vi "Joystick Get.vi"() -> (0 "Raw Joystick 2 Data":T2, 1 "Raw Joystick 1 Data":T2, 3 "Mapped Data":T3)   [LabVIEW 2013]
uses:
  Joystick Data.ctl
  <vilib>/Rock Robotics/WPI/Joystick/WPI_JoystickButtonState.ctl
  <vilib>/Rock Robotics/WPI/Joystick/WPI_JoystickGetSetRefNum.vi
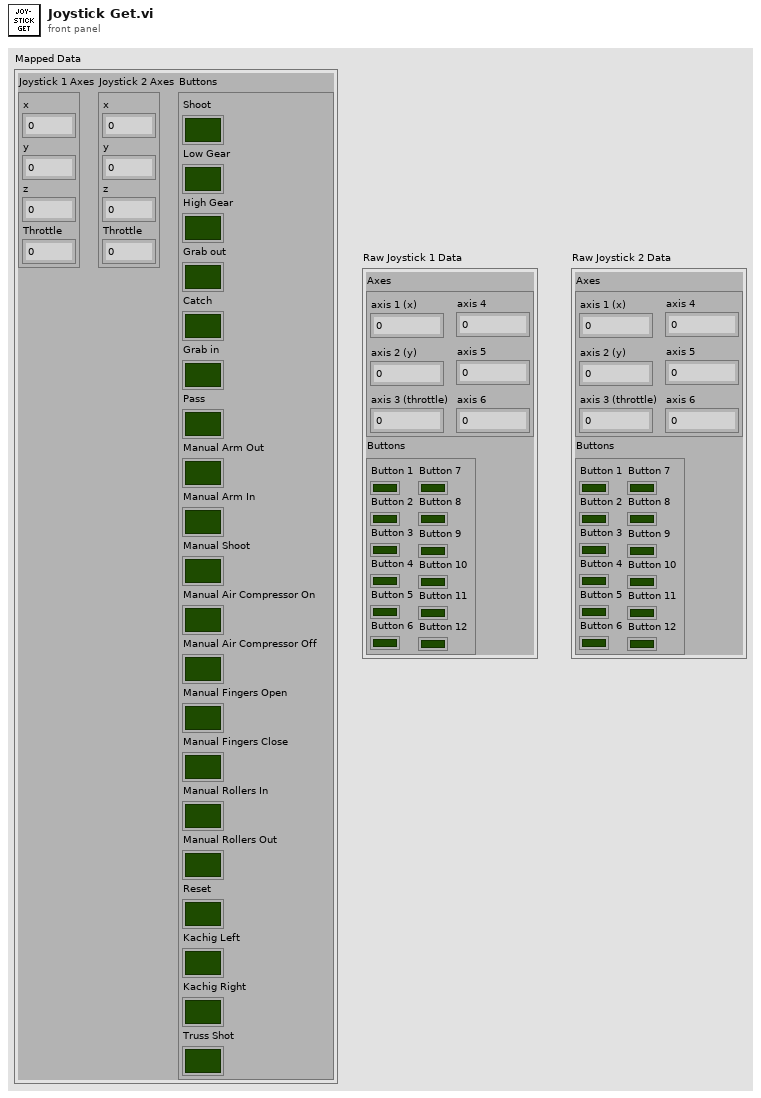
[diagram p1: front panel]
types:
  T1 = typedef "WPI_JoystickButtonState.ctl" = cluster{"Button 1":bool, "Button 2":bool, "Button 3":bool, "Button 4":bool, "Button 5":bool, "Button 6":bool, "Button 7":bool, "Button 8":bool, "Button 9":bool, "Button 10":bool, "Button 11":bool, "Button 12":bool}
  T2 = cluster{"Axes":cluster{"axis 1 (x)":dbl, "axis 2 (y)":dbl, "axis 3 (throttle)":dbl, "axis 4":dbl, "axis 5":dbl, "axis 6":dbl}, "Buttons":T1}
  T3 = typedef "Joystick Data.ctl" = cluster{"Joystick 1 Axes":cluster{"x":dbl, "y":dbl, "z":dbl, "Throttle":dbl}, "Joystick 2 Axes":cluster{"x":dbl, "y":dbl, "z":dbl, "Throttle":dbl}, "Buttons":cluster{"Shoot":bool, "Low Gear":bool, "High Gear":bool, "Grab out":bool, "Catch":bool, "Grab in":bool, "Pass":bool, "Manual Arm Out":bool, "Manual Arm In":bool, "Manual Shoot":bool, "Manual Air Compressor On":bool, "Manual Air Compressor Off":bool, "Manual Fingers Open":bool, "Manual Fingers Close":bool, "Manual Rollers In":bool, "Manual Rollers Out":bool, "Reset":bool, "Kachig Left":bool, "Kachig Right":bool, "Truss Shot":bool}}
  T4 = typedef "WPI_JoystickDevRef.ctl" = cluster{"Device":T5}
  T5 = typedef "WPI_JoystickDeviceEnum.ctl" = enum16{"USB 1", "USB 2", "USB 3", "USB 4", "Kinect 1", "Kinect 2"}
  T6 = cluster{"axis 1 (x)":dbl, "axis 2 (y)":dbl, "axis 3 (throttle)":dbl, "axis 4":dbl, "axis 5":dbl, "axis 6":dbl}
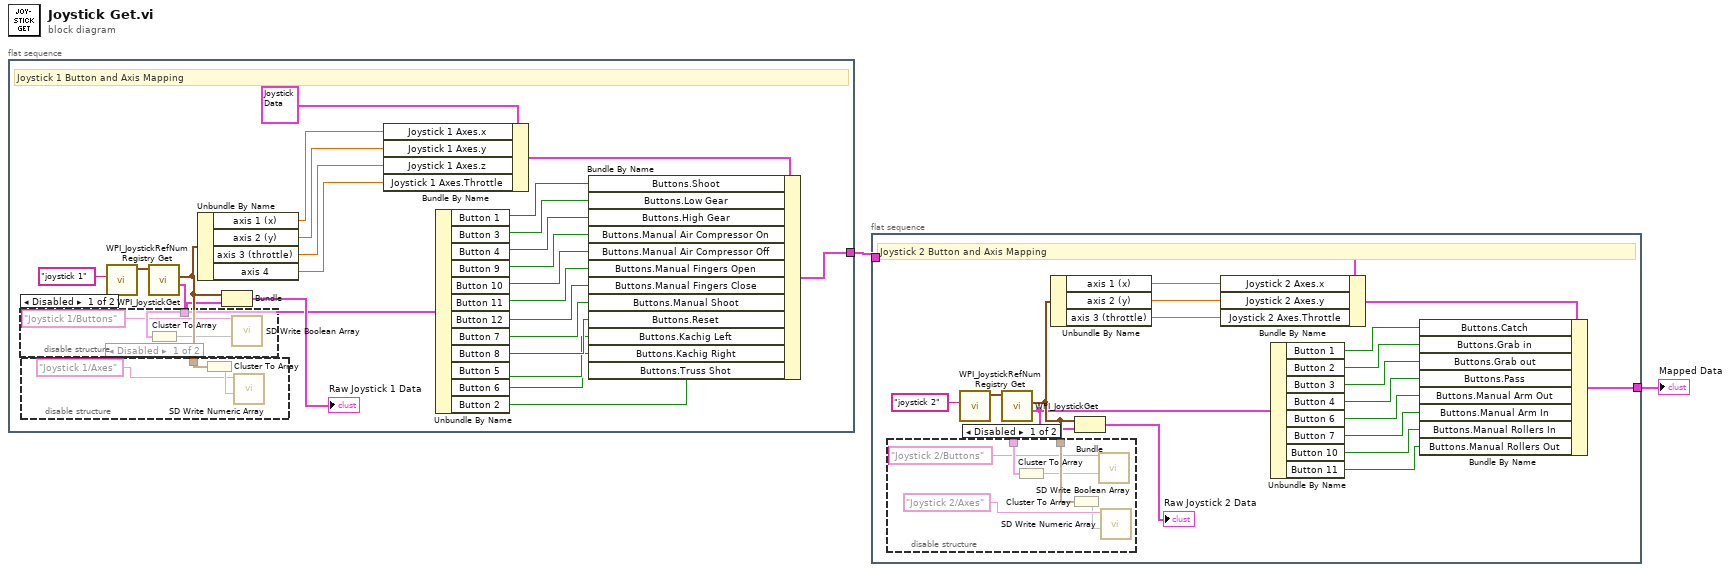
[diagram p0: block diagram]
diagram:
  n1 = flat-sequence {
    tunnel: [w24] -> w2
    frame #0 {
      # "Joystick 1 Button and Axis Mapping"
      n2 = call <vilib>:"WPI_JoystickRefNum Registry Get.vi"("refnum name"="joystick 1") -> ("JoystickDevRef"=w25:T4)  [unwired: 9 in, 1 out]
      n3 = call <vilib>:"WPI_JoystickGet.vi"("JoystickDevRef"=w25) -> ("Buttons"=w6:T1, "Axes"=w7:T6)  [unwired: 4 in, 1 out]
      n4 = disable-structure shown="Disabled" {
        disable-tunnel: w6 -> [w29 _]
        frame Disabled {
          n5 = Cluster To Array(cluster=w29) -> (array=w28:bool[])
          n6 = call <vilib>:"SD Write Boolean Array.vi"("Boolean Array"=w28, "Name"="Joystick 1/Buttons" ("refnum name")) -> ()  [unwired: 8 in, 2 out]
        }
        frame Enabled {
        }
      }
      n7 = disable-structure shown="Disabled" {
        disable-tunnel: w7 -> [w32 _]
        frame Disabled {
          n8 = Cluster To Array(cluster=w32) -> (array=w31:dbl[])
          n9 = call <vilib>:"SD Write Numeric Array.vi"("Numeric Array"=w31, "Name"="Joystick 1/Axes" ("refnum name")) -> ()  [unwired: 8 in, 2 out]
        }
        frame Enabled {
        }
      }
      n10 = Unbundle By Name(w7) -> ("axis 1 (x)"=w15:dbl, "axis 2 (y)"=w14:dbl, "axis 3 (throttle)"=w13:dbl, "axis 4"=w12:dbl)
      n11 = Bundle("Axes"=w7, "Buttons"=w6) -> (→"Raw Joystick 1 Data":T2)  [unwired: 1 in]
      n12 = Bundle By Name(cluster=T3 {"Joystick 1 Axes"={"x"=0.0, "y"=0.0, "z"=0.0, "Throttle"=0.0}, "Joystick 2 Axes"={"x"=0.0, "y"=0.0, "z"=0.0, "Throttle"=0.0}, "Buttons"={"Shoot"=FALSE, "Low Gear"=FALSE, "High Gear"=FALSE, "Grab out"=FALSE, "Catch"=FALSE, "Grab in"=FALSE, "Pass"=FALSE, "Manual Arm Out"=FALSE, "Manual Arm In"=FALSE, "Manual Shoot"=FALSE, "Manual Air Compressor On"=FALSE, "Manual Air Compressor Off"=FALSE, "Manual Fingers Open"=FALSE, "Manual Fingers Close"=FALSE, "Manual Rollers In"=FALSE, "Manual Rollers Out"=FALSE, "Reset"=FALSE, "Kachig Left"=FALSE, "Kachig Right"=FALSE, "Truss Shot"=FALSE}} ("output cluster"), "Joystick 1 Axes.x"=w15, "Joystick 1 Axes.y"=w14, "Joystick 1 Axes.z"=w13, "Joystick 1 Axes.Throttle"=w12) -> (w11:T3)
      n13 = Unbundle By Name(w6) -> ("Button 1"=w23:bool, "Button 3"=w22:bool, "Button 4"=w21:bool, "Button 9"=w20:bool, "Button 10"=w19:bool, "Button 11"=w18:bool, "Button 12"=w17:bool, "Button 7"=w16:bool, "Button 8"=w9:bool, "Button 5"=w5:bool, "Button 6"=w4:bool, "Button 2"=w3:bool)
      n14 = Bundle By Name(cluster=w11, "Buttons.Shoot"=w23, "Buttons.Low Gear"=w22, "Buttons.High Gear"=w21, "Buttons.Manual Air Compressor On"=w20, "Buttons.Manual Air Compressor Off"=w19, "Buttons.Manual Fingers Open"=w18, "Buttons.Manual Fingers Close"=w17, "Buttons.Manual Shoot"=w16, "Buttons.Reset"=w9, "Buttons.Kachig Left"=w5, "Buttons.Kachig Right"=w4, "Buttons.Truss Shot"=w3) -> (w24:T3)
    }
  }
  n15 = flat-sequence {
    tunnel: w2 -> [w39]
    tunnel: [w49] -> w1
    frame #0 {
      # "Joystick 2 Button and Axis Mapping"
      n16 = call <vilib>:"WPI_JoystickRefNum Registry Get.vi"("refnum name"="joystick 2") -> ("JoystickDevRef"=w50:T4)  [unwired: 9 in, 1 out]
      n17 = call <vilib>:"WPI_JoystickGet.vi"("JoystickDevRef"=w50) -> ("Buttons"=w33:T1, "Axes"=w34:T6)  [unwired: 4 in, 1 out]
      n18 = disable-structure shown="Disabled" {
        disable-tunnel: w34 -> [w57 _]
        disable-tunnel: w33 -> [w56 _]
        frame Disabled {
          n19 = Cluster To Array(cluster=w56) -> (array=w54:bool[])
          n20 = Cluster To Array(cluster=w57) -> (array=w52:dbl[])
          n21 = call <vilib>:"SD Write Boolean Array.vi"("Boolean Array"=w54, "Name"="Joystick 2/Buttons" ("refnum name")) -> ()  [unwired: 8 in, 2 out]
          n22 = call <vilib>:"SD Write Numeric Array.vi"("Numeric Array"=w52, "Name"="Joystick 2/Axes" ("refnum name")) -> ()  [unwired: 8 in, 2 out]
        }
        frame Enabled {
        }
      }
      n23 = Unbundle By Name(w34) -> ("axis 1 (x)"=w42:dbl, "axis 2 (y)"=w41:dbl, "axis 3 (throttle)"=w40:dbl)
      n24 = Bundle("Axes"=w34, "Buttons"=w33) -> (→"Raw Joystick 2 Data":T2)  [unwired: 1 in]
      n25 = Bundle By Name(cluster=w39, "Joystick 2 Axes.x"=w42, "Joystick 2 Axes.y"=w41, "Joystick 2 Axes.Throttle"=w40) -> (w38:T3)
      n26 = Unbundle By Name(w33) -> ("Button 1"=w48:bool, "Button 2"=w37:bool, "Button 3"=w36:bool, "Button 4"=w47:bool, "Button 6"=w46:bool, "Button 7"=w45:bool, "Button 10"=w44:bool, "Button 11"=w43:bool)
      n27 = Bundle By Name(cluster=w38, "Buttons.Catch"=w48, "Buttons.Grab in"=w37, "Buttons.Grab out"=w36, "Buttons.Pass"=w47, "Buttons.Manual Arm Out"=w46, "Buttons.Manual Arm In"=w45, "Buttons.Manual Rollers In"=w44, "Buttons.Manual Rollers Out"=w43) -> (w49:T3)
    }
  }
  "Mapped Data" <- w1
